vi "TakeVideoTest.vi"() -> ()   [LabVIEW 2018]
uses:
  Andor SDK/Copy of Andor SDK.lvlib
panel:
  out "3":u32
  out "2":u32
  out "1":u32
  out "0":u32
  out "Average Delay [ms]":dbl format="%#_3f"
  in  "stop":bool
  out "Return from Get Acquisition":u32=20002
  out "Intensity Graph":i32[][](graph)
  out "Return from GetStatus":u32=73
  out "Return from Start Acquisition":u32=20002
  in  "vend":i32=512
  in  "vstart":i32=1
  in  "hend":i32=512
  in  "hstart":i32=1
  in  "Set Exposure Time [s]":sgl=0.1 format="%.2f"
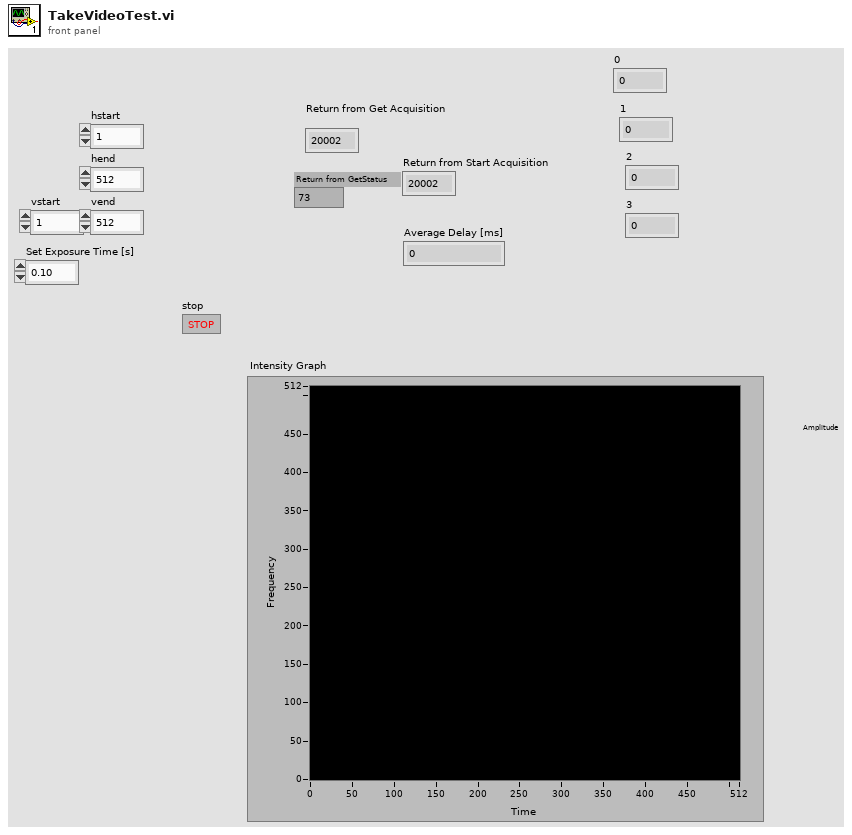
[diagram p1: front panel]
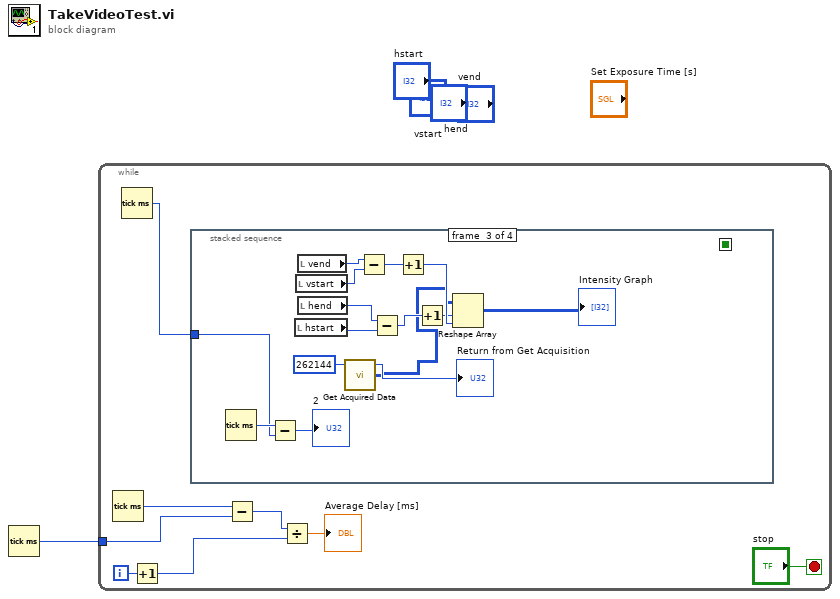
[diagram p0: block diagram]
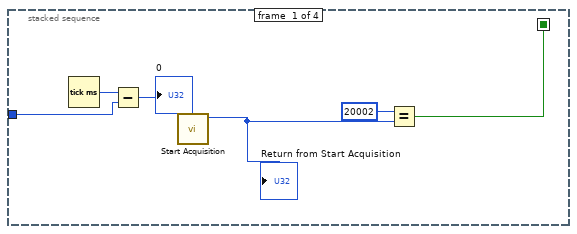
[diagram p2: hidden frame]
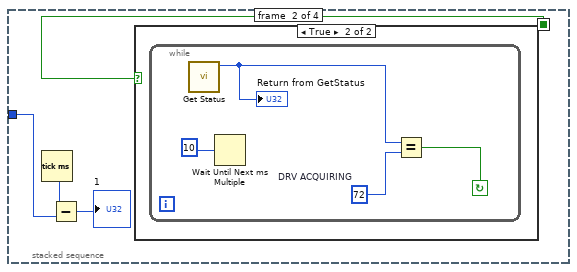
[diagram p3: hidden frame]
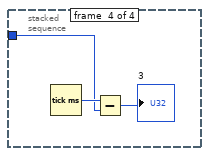
[diagram p5: hidden frame]
diagram:
  n1 = Tick Count (ms)() -> (millisecond timer value=w1:u32)
  n2 = while {
    tunnel: w1 -> [w7]
    i -> [w6]
    stop <- "stop" stop-if-true
    n3 = Tick Count (ms)() -> (millisecond timer value=w8:u32)
    n4 = Tick Count (ms)() -> (millisecond timer value=w2:u32)
    n5 = Increment(x=w6) -> (x+1=w3:i32)
    n6 = stacked-sequence {
      seq-local: [w15 _ _ _] -> [_ w19 _ _]
      tunnel: w2 -> [w11 w16 w27 w39]
      frame #0 {
        n7 = Tick Count (ms)() -> (millisecond timer value=w12:u32)
        n8 = Subtract(x=w12, y=w11) -> (x-y=→"0":u32)
        n9 = call "Start Acquisition.vi"() -> ("function return"=w14:u32)  [unwired: 11 in]
        "Return from Start Acquisition" <- w14
        n10 = Equal?(x=u32 20002, y=w14) -> (x = y?=w15:bool)
      }
      frame #1 {
        n11 = Tick Count (ms)() -> (millisecond timer value=w18:u32)
        n12 = Subtract(x=w18, y=w16) -> (x-y=→"1":u32)
        n13 = case shown="True" w19 {
          frame False {
          }
          frame True {
            n14 = while {
              stop <- w22 continue-if-true
              w21 = u16 72  # DRV ACQUIRING
              n15 = call "Get Status.vi"() -> ("status out"=w20:i32)  [unwired: 10 in, 1 out]
              "Return from GetStatus" <- w20
              n16 = Wait Until Next ms Multiple(millisecond multiple=u32 10) -> ()  [unwired: 1 out]
              n17 = Equal?(x=w20, y=w21) -> (x = y?=w22:bool)
            }
          }
        }
      }
      frame #2 {
        n18 = Tick Count (ms)() -> (millisecond timer value=w29:u32)
        n19 = Subtract(x=w29, y=w27) -> (x-y=→"2":u32)
        n20 = local read "hstart"() -> (w34:i32)
        n21 = local read "vstart"() -> (w36:i32)
        n22 = local read "vend"() -> (w37:i32)
        n23 = local read "hend"() -> (w35:i32)
        n24 = call "Get Acquired Data.vi"("size"=u32 262144) -> ("arr 2"=w24:i32[][], "function return"=→"Return from Get Acquisition":u32)  [unwired: 3 in]
        n25 = Subtract(x=w37, y=w36) -> (x-y=w33:i32)
        n26 = Subtract(x=w35, y=w34) -> (x-y=w32:i32)
        n27 = Increment(x=w33) -> (x+1=w31:i32)
        n28 = Increment(x=w32) -> (x+1=w30:i32)
        n29 = Reshape Array(w24, w30, w31) -> (→"Intensity Graph":i32[][])
      }
      frame #3 {
        n30 = Tick Count (ms)() -> (millisecond timer value=w41:u32)
        n31 = Subtract(x=w41, y=w39) -> (x-y=→"3":u32)
      }
    }
    n32 = Subtract(x=w8, y=w7) -> (x-y=w4:u32)
    n33 = Divide(x=w4, y=w3) -> (x/y=→"Average Delay [ms]":dbl)
  }
